vi "HIOKI PW3390 Continuous Acquisition Integrarion.vi"() -> ()   [LabVIEW 2009]
doc: "Starting this program starts integration, and stopping this program stops integration. During running, the specified measurement data are output in 100ms cycle. Restarting this program leads reset and restart integration."
uses:
  <instrlib>/PW3390/Common/_Initialize/HIOKI PW3390 Initialize LAN.vi
  <instrlib>/PW3390/Common/_Initialize/HIOKI PW3390 Initialize RS-232C.vi
panel:
  out "Selected Item out":string[](array[string])
  out "Data out":dbl[](array[numeric])
  in  "Item":T1(array[cluster])=[{"Item"=enum."IH", "Ch(0:Ch1)"=enum."1"}, {"Item"=enum."WP+", "Ch(0:Ch1)"=enum."1"}, {"Item"=enum."WP-", "Ch(0:Ch1)"=enum."1"}, {"Item"=enum."WP", "Ch(0:Ch1)"=enum."1"}, {"Item"=enum."Laptime", "Ch(0:Ch1)"=enum."1"}, {"Item"=enum."Laptime(ms)", "Ch(0:Ch1)"=enum."1"}]
  out "error out":errorcluster={"status"=FALSE, "code"=1073676293, "source"="VISA読み取り/HIOKI PW3390 Read_Write.vi->HIOKI PW3390 ESR.vi->HIOKI PW3390 Meas Integ Stop.vi->HIOKI PW3390 Continuous Acquisition Integrarion.vi"}
  in  "Communication Interface":enum16{"LAN", "RS-232C"}(ring)
  in  "COM Port":refnum<visa-resource-name>="COM1"
  in  "baud rate (38400bps)":u32=38400
  in  "IP Address":string="192.168.1.1"
  in  "Stop":bool
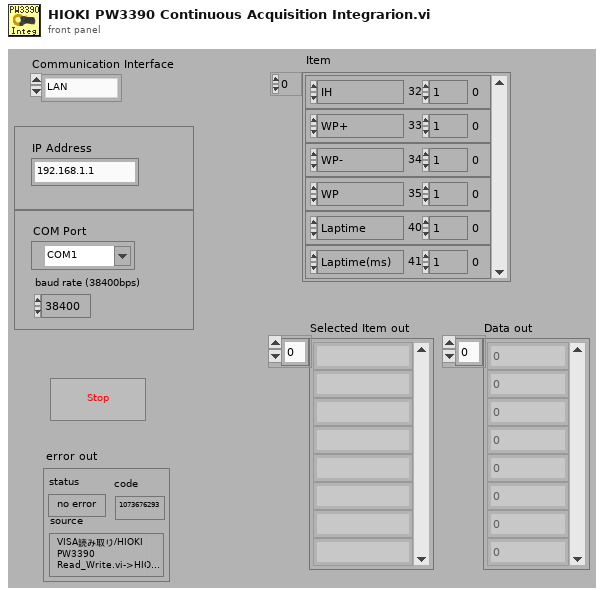
[diagram p1: front panel]
types:
  T1 = cluster{"Item":enum16{"Urms", "Umn", "Uac", "Udc", "Ufnd", "Upk+", "Upk-", "Uthd", "Urf", "Uunb", "Irms", "Imn", "Iac", "Idc", "Ifnd", "Ipk+", "Ipk-", "Ithd", "Irf", "Iunb", "P", "S", "Q", "PF", "DEG U", "DEG I", "DEG P", "f", "EFFI", "LOSS", "IH+", "IH-", "IH", "WP+", "WP-", "WP", "CH A", "CH B", "Pm", "Slip", "Laptime", "Laptime(ms)"}, "Ch(0:Ch1)":enum16{"1", "2", "3", "4", "12", "34", "123"}}[]
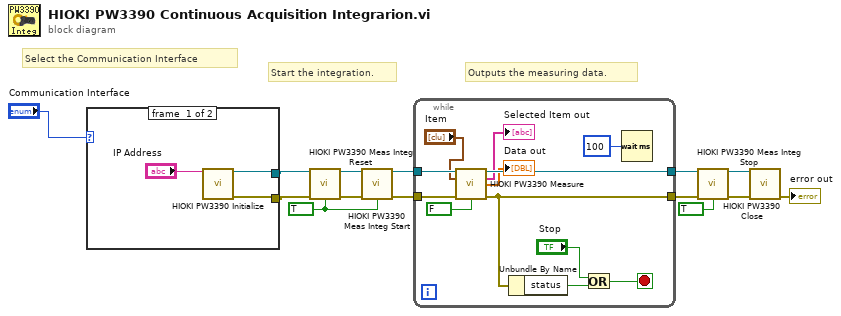
[diagram p0: block diagram]
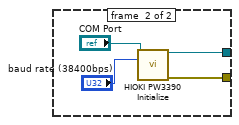
[diagram p2: hidden frame]
diagram:
  w2 = TRUE ("Error Out (F: Off)")
  # "Select the Communication Interface"
  # "Outputs the measuring data."
  # "Start the integration."
  n1 = case shown="\"LAN\", デフォルト" "Communication Interface" {
    tunnel: [w16 w21] -> w4
    tunnel: [w15 w20] -> w5
    frame #0 {
      n2 = call-poly <instrlib>:"HIOKI PW3390 Initialize.vi"("IP Address"="IP Address") -> ("VISA Resource out"=w16:refnum<visa-resource-name>, "error out"=w15:errorcluster)  [unwired: 12 in, 1 out]
    }
    frame #1 {
      n3 = call-poly <instrlib>:"HIOKI PW3390 Initialize.vi"("COM Port"="COM Port", "baud rate (38400bps)"="baud rate (38400bps)") -> ("VISA Resource out"=w21:refnum<visa-resource-name>, "error out"=w20:errorcluster)  [unwired: 11 in, 1 out]
    }
  }
  n4 = call <instrlib>:"HIOKI PW3390 Meas Integ Reset.vi"("VISA Resource"=w4, "error in (no error)"=w5, "Error Out (F: Off)"=w2) -> ("VISA Resource out"=w8:refnum<visa-resource-name>, "error out"=w7:errorcluster)  [unwired: 11 in]
  n5 = call <instrlib>:"HIOKI PW3390 Meas Integ Start.vi"("VISA Resource"=w8, "error in (no error)"=w7, "Error Out (F: Off)"=w2) -> ("VISA Resource out"=w14:refnum<visa-resource-name>, "error out"=w13:errorcluster)  [unwired: 11 in]
  n6 = while {
    tunnel: w14 -> [w33]
    tunnel: w13 -> [w32]
    tunnel: [w31] -> w12
    tunnel: [w27] -> w10
    stop <- w28 stop-if-true
    n7 = call <instrlib>:"HIOKI PW3390 Measure.vi"("VISA Resource"=w33, "Item"="Item", "error in (no error)"=w32, "Error Out (F: Off)"=FALSE) -> ("VISA Resource out"=w31:refnum<visa-resource-name>, "Selected Item out"=→"Selected Item out":string[], "Data out"=→"Data out":dbl[], "error out"=w27:errorcluster)  [unwired: 6 in, 2 out]
    n8 = Unbundle By Name(w27) -> ("status"=w26:bool)
    n9 = Or(x="Stop", y=w26) -> (x .or. y?=w28:bool)
    n10 = Wait (ms)(milliseconds to wait=u32 100) -> ()  [unwired: 1 out]
  }
  n11 = call <instrlib>:"HIOKI PW3390 Meas Integ Stop.vi"("VISA Resource"=w12, "error in (no error)"=w10, "Error Out (F: Off)"=TRUE) -> ("VISA Resource out"=w11:refnum<visa-resource-name>, "error out"=w9:errorcluster)  [unwired: 11 in]
  n12 = call <instrlib>:"HIOKI PW3390 Close.vi"("VISA Resource"=w11, "error in (no error)"=w9) -> ("error out"=→"error out":errorcluster)  [unwired: 13 in]
